vi "SubPanel - Voltages and Currents Analysis.vi"(8 "error in":errorcluster, 10 "Samples per Channel":i32, 11 "Message FPGA":T1) -> (0 "error out":errorcluster)   [LabVIEW 2021]
uses:
  Typedefs/Signal Parameters.ctl
  Typedefs/Message FPGA.ctl
panel:
  in  "Phases Parameters":enum32{"Phase 1", "Phase 2", "Phase 3"}(tab)
  out "Phase 1 Voltage":T2
  out "Phase 1 Current":T2
  out "Phase 2 Current":T2
  out "Phase 2 Voltage":T2
  out "Phase 3 Current":T2
  out "Phase 3 Voltage":T2
  in  "L3 Voltage":bool=TRUE caption="Checkbox"
  in  "L3 Current":bool=TRUE caption="Checkbox"
  in  "L2 Voltage":bool=TRUE caption="Checkbox"
  in  "L2 Current":bool=TRUE caption="Checkbox"
  in  "L1 Voltage":bool=TRUE caption="Checkbox"
  in  "L1 Current":bool=TRUE caption="Checkbox"
  out "Voltages and Currents Chart":dbl[][](graph) caption="Waveform Chart - Dark"
  # "Visible Signals"
  # "Signals Parameters"
  # "Voltage"
  # "Current"
  # "Voltage"
  # "Current"
  # "Voltage"
  # "Current"
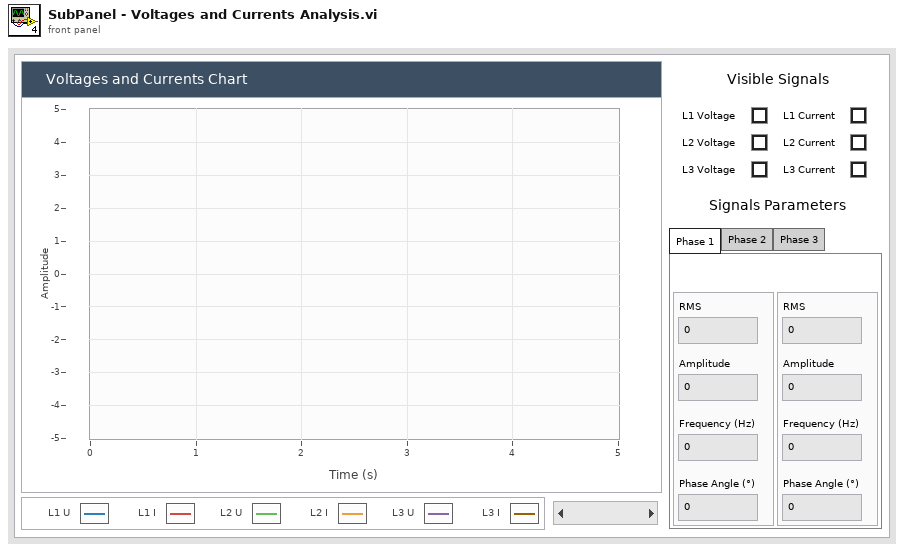
[diagram p1: front panel]
types:
  T1 = typedef "Message FPGA.ctl" = cluster{"Channel 1 Data (L1 U)":dbl[], "Channel 2 Data (L1 I)":dbl[], "Channel 3 Data (L2 U)":dbl[], "Channel 4 Data (L2 I)":dbl[], "Channel 5 Data (L3 U)":dbl[], "Channel 6 Data (L3 I)":dbl[]}
  T2 = typedef "Signal Parameters.ctl" = cluster{"RMS":dbl, "Amplitude":dbl, "Frequency (Hz)":dbl, "Phase Angle (°)":dbl}
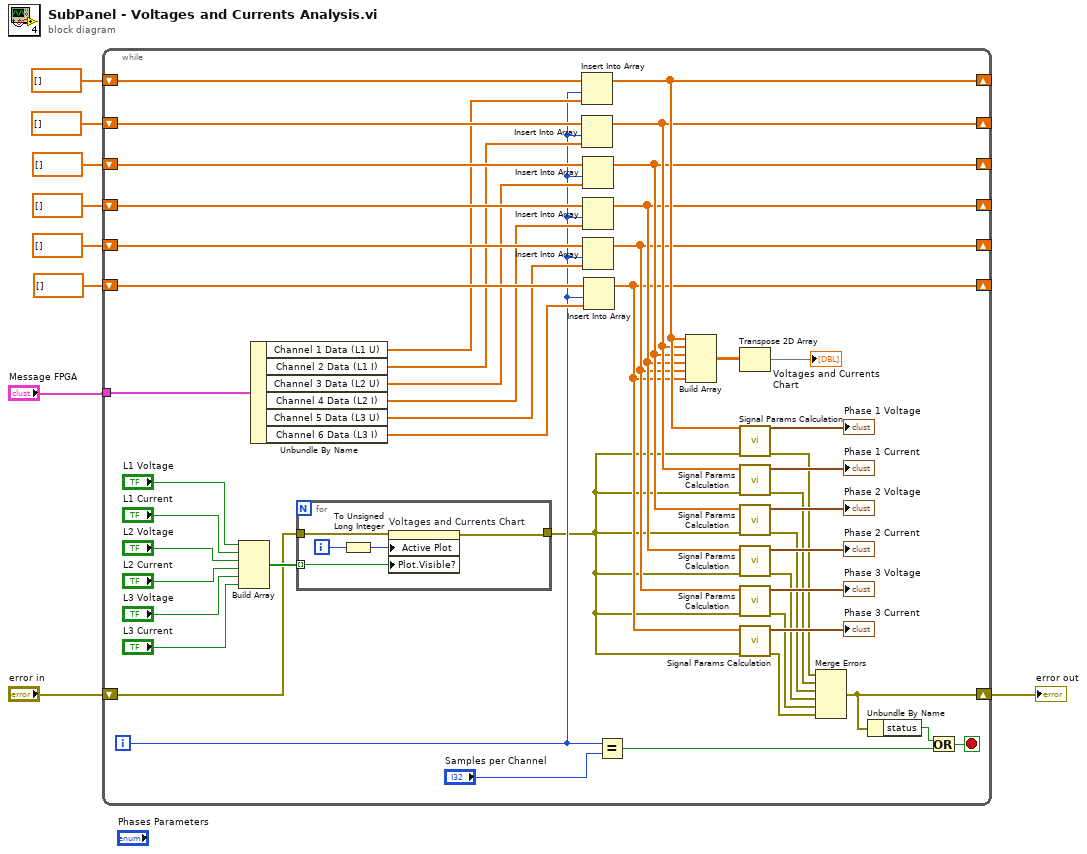
[diagram p0: block diagram]
diagram:
  n1 = while {
    tunnel: "Message FPGA" -> [w57]
    shift-right: [w40] -> _
    shift-left: dbl[] [] -> [w56]
    shift-right: [w39] -> _
    shift-left: dbl[] [] -> [w55]
    shift-right: [w38] -> _
    shift-left: dbl[] [] -> [w54]
    shift-right: [w37] -> _
    shift-left: dbl[] [] -> [w53]
    shift-right: [w36] -> _
    shift-left: dbl[] [] -> [w52]
    shift-right: [w35] -> _
    shift-left: dbl[] [] -> [w51]
    shift-right: [w20] -> w1
    shift-left: "error in" -> [w21]
    i -> [w42]
    stop <- w19 stop-if-true
    n2 = Build Array("L1 Voltage", "L1 Current", "L2 Voltage", "L2 Current", "L3 Voltage", "L3 Current") -> (w29:bool[])
    n3 = Unbundle By Name(w57) -> ("Channel 1 Data (L1 U)"=w50:dbl[], "Channel 2 Data (L1 I)"=w49:dbl[], "Channel 3 Data (L2 U)"=w48:dbl[], "Channel 4 Data (L2 I)"=w47:dbl[], "Channel 5 Data (L3 U)"=w46:dbl[], "Channel 6 Data (L3 I)"=w45:dbl[])
    n4 = for {
      tunnel: w29 -> [w60] mode=indexing
      tunnel: w21 -> [w59]
      tunnel: [w58] -> w10
      i -> [w62]
      n5 = To Unsigned Long Integer(number=w62) -> (unsigned 32bit integer=w61:u32)
      n6 = property on="Voltages and Currents Chart" class="WFChart (strict)"(error in=w59, "Active Plot"=w61, "Plot.Visible?"=w60) -> (error out=w58:errorcluster)  [unwired: 1 in, 1 out]
    }
    n7 = Insert Into Array(array=w56, index=w42, new element=w50) -> (w40:dbl[])
    n8 = Insert Into Array(array=w55, index=w42, new element=w49) -> (w39:dbl[])
    n9 = Insert Into Array(array=w54, index=w42, new element=w48) -> (w38:dbl[])
    n10 = Insert Into Array(array=w53, index=w42, new element=w47) -> (w37:dbl[])
    n11 = Insert Into Array(array=w52, index=w42, new element=w46) -> (w36:dbl[])
    n12 = Insert Into Array(array=w51, index=w42, new element=w45) -> (w35:dbl[])
    n13 = Equal?(x=w42, y="Samples per Channel") -> (x = y?=w17:bool)
    n14 = Build Array(w40, w39, w38, w37, w36, w35) -> (w43:dbl[][])
    n15 = Transpose 2D Array(2D array=w43) -> (transposed array=→"Voltages and Currents Chart":dbl[][])
    n16 = call "Signal Params Calculation.vi"("error in"=w10, "Signal"=w40) -> ("error out"=w11:errorcluster, "Signal Parameters"=→"Phase 1 Voltage":T2)  [unwired: 8 in]
    n17 = call "Signal Params Calculation.vi"("error in"=w10, "Signal"=w39) -> ("error out"=w12:errorcluster, "Signal Parameters"=→"Phase 1 Current":T2)  [unwired: 8 in]
    n18 = call "Signal Params Calculation.vi"("error in"=w10, "Signal"=w38) -> ("error out"=w13:errorcluster, "Signal Parameters"=→"Phase 2 Voltage":T2)  [unwired: 8 in]
    n19 = call "Signal Params Calculation.vi"("error in"=w10, "Signal"=w37) -> ("error out"=w14:errorcluster, "Signal Parameters"=→"Phase 2 Current":T2)  [unwired: 8 in]
    n20 = call "Signal Params Calculation.vi"("error in"=w10, "Signal"=w36) -> ("error out"=w15:errorcluster, "Signal Parameters"=→"Phase 3 Voltage":T2)  [unwired: 8 in]
    n21 = call "Signal Params Calculation.vi"("error in"=w10, "Signal"=w35) -> ("error out"=w16:errorcluster, "Signal Parameters"=→"Phase 3 Current":T2)  [unwired: 8 in]
    n22 = Merge Errors(w11, w12, w13, w14, w15, w16) -> (w20:errorcluster)
    n23 = Unbundle By Name(w20) -> ("status"=w18:bool)
    n24 = Or(x=w18, y=w17) -> (x .or. y?=w19:bool)
  }
  "error out" <- w1
